vi "ProcessingFrame.vi"(8 "error in (no error)":errorcluster, 11 "navX - Base in":refnum<class "navX - I2C.lvclass">) -> (0 "error out":errorcluster, 3 "navX - Base out":refnum<class "navX - I2C.lvclass">)   [LabVIEW 2015, in "navX Library v3.lvlib" / "navX - I2C.lvclass"]
uses:
  navX - I2C.lvclass
  navX - I2C.lvclass/navX - I2C.ctl
  navX - Interface/navX - Interface.lvclass/navX - Interface.ctl
  navX - Interface/navX - Interface.lvclass
  navX Registry Cache/navX Registry Cache.lvclass
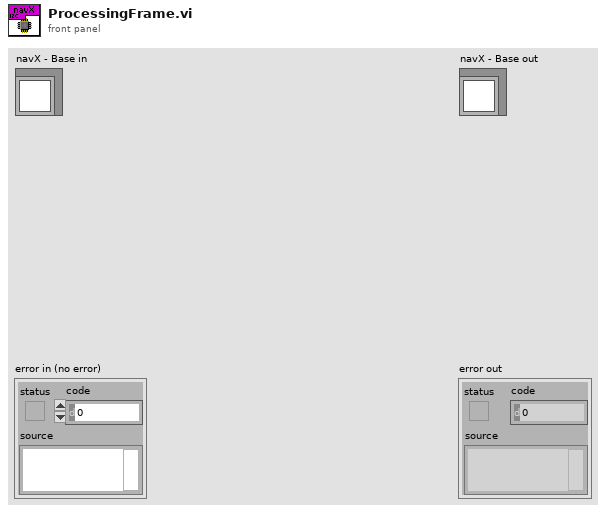
[diagram p1: front panel]
types:
  T1 = typedef "WPI_I2CDevRef.ctl" = cluster{"DevStatus":errorcluster, "Device Address":u8, "Handle":i32, "I2C Bus":T2}
  T2 = typedef "i2c_bus.ctl" = enum16{"I2C On-Board", "I2C MXP", "Invalid"}
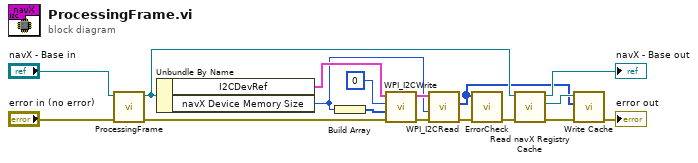
[diagram p0: block diagram]
diagram:
  n1 = call-parent "ProcessingFrame.vi"("error in (no error)"="error in (no error)", "navX - Interface in"="navX - Base in") -> ("error out"=w6:errorcluster, "navX - Interface out"=w11:refnum<class "navX - I2C.lvclass">)  [unwired: 8 in]
  n2 = Unbundle By Name(w11) -> ("I2CDevRef"=w5:T1, "navX Device Memory Size"=w4:i32)
  n3 = Build Array(w4) -> (w7:i32[])
  n4 = call <vilib>:"WPI_I2CWrite.vi"("error in (no error)"=w6, "I2CDataToSend"=w7, "I2CRegister"=u8 0 ("hex"), "I2CDevRef"=w5) -> ("error out"=w10:errorcluster, "I2CDevRef"=w9:T1)  [unwired: 6 in]
  n5 = call <vilib>:"WPI_I2CRead.vi"("error in (no error)"=w10, "I2CBytesToRead"=w4, "I2CDevRef"=w9) -> ("error out"=w3:errorcluster, "Data Out"=w2:u8[])  [unwired: 6 in, 1 out]
  n6 = call "ErrorCheck.vi"("error in (no error)"=w3, "I2C Data in"=w2) -> ("error out"=w1:errorcluster)  [unwired: 9 in]
  n7 = call "Read navX Registry Cache.vi"("error in (no error)"=w1, "navX - Interface in"=w11) -> ("error out"=w14:errorcluster, "navX Library v3.lvlib:navX Registry Cache.lvclass"=w15:refnum<class "navX Registry Cache.lvclass">, "navX - Interface out"=→"navX - Base out":refnum<class "navX - I2C.lvclass">)  [unwired: 7 in]
  n8 = call "Write Cache.vi"("error in (no error)"=w14, "Registry Cache in"=w2, "navX Registry Cache in"=w15) -> ("error out"=→"error out":errorcluster)  [unwired: 7 in, 1 out]
